vi "ShooterPID.vi"(9 "Shooter Refnum 2":string="My Motor RefNum", 10 "Shooter Refnum 1":string="My Motor RefNum") -> ()   [LabVIEW 2019]
uses:
  <vilib>/Rock Robotics/WPI/ThirdParty/REV Robotics/SPARK MAX/Typedef/Spark MAX Control Type.ctl
  sensors.vi
panel:
  in  "Setpoint Changer":dbl
  in  "Setpoint":dbl(slide) scale=-5700.0..5700.0
  out "PID Chart":T1(graph)
  in  "PID Constants":T2={"P Gain"=0.0012, "I Gain"=1e-06, "D Gain"=0.012, "F Gain"=0.00023, "I Zone"=100.0, "Min Output"=-1.0, "Max Output"=1.0} {"Max Output" min=-1.0 max=1.0 step=0.01; "Min Output" min=-1.0 max=1.0 step=0.01; "I Zone" step=0.01; "F Gain" step=0.01; "D Gain" step=0.01; "I Gain" step=0.01; "P Gain" min=0.0 step=0.01}
  in  "PID Constants 2":T2={"P Gain"=0.0012, "I Gain"=1e-06, "D Gain"=0.012, "F Gain"=0.00023, "I Zone"=100.0, "Min Output"=-1.0, "Max Output"=1.0} {"Max Output" min=-1.0 max=1.0 step=0.01; "Min Output" min=-1.0 max=1.0 step=0.01; "I Zone" step=0.01; "F Gain" step=0.01; "D Gain" step=0.01; "I Gain" step=0.01; "P Gain" min=0.0 step=0.01}
  out "PID Chart 2":T1(graph)
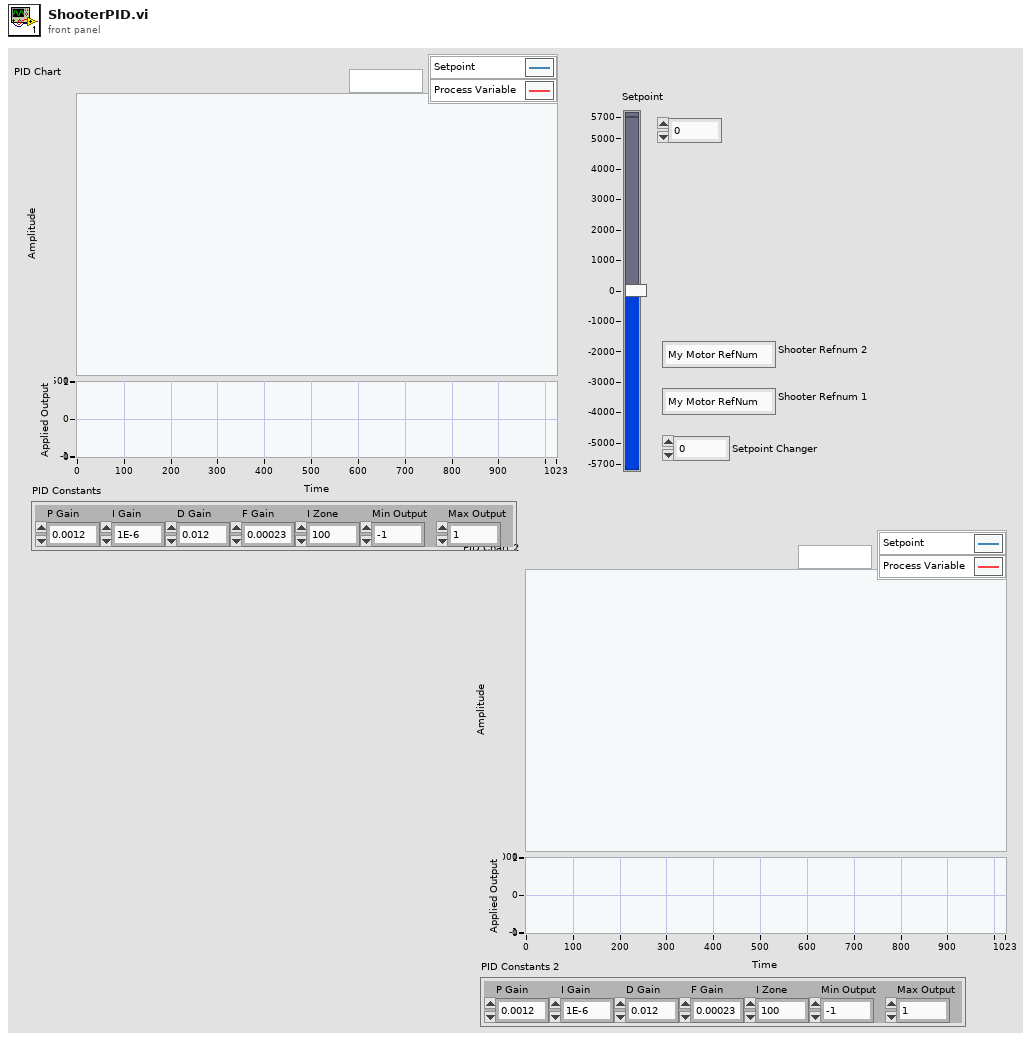
[diagram p1: front panel]
types:
  T1 = cluster{"Sensor Velocity":dbl, "Setpoint":dbl, "Applied Output":dbl}
  T2 = cluster{"P Gain":dbl, "I Gain":dbl, "D Gain":dbl, "F Gain":dbl, "I Zone":dbl, "Min Output":dbl, "Max Output":dbl}
  T3 = typedef "WPI_MotorControlDeviceRef.ctl" = cluster{"DeviceStatus":errorcluster, "Type":T4, "PWM":cluster{"PWM Channel":T5, "DeadBand":T6}, "CAN":cluster{"Device Number":u8, "SetOutput VI Ref":variant, "GetOutput VI Ref":variant, "Enable VI Ref":variant, "Disable VI Ref":variant, "Data":variant}, "Invert":bool, "DIO PWM":cluster{"PWM \"Enable\" Channel":T5, "DIOChannel":T7, "PWM Rate":dbl}}
  T4 = typedef "WPI_MotorControlType.ctl" = enum16{"PWM", "CAN", "DIO PWM"}
  T5 = typedef "FPGA_DIOPWMChannel.ctl" = enum8{"PWM 0", "PWM 1", "PWM 2", "PWM 3", "PWM 4", "PWM 5", "PWM 6", "PWM 7", "PWM 8", "PWM 9", "PWM MXP 0", "PWM MXP 1", "PWM MXP 2", "PWM MXP 3", "PWM MXP 4", "PWM MXP 5", "PWM MXP 6", "PWM MXP 7", "PWM MXP 8", "PWM MXP 9", "Invalid"}
  T6 = typedef "WPI_PWMDeadband.ctl" = cluster{"Name":string, "maxPositivePwm":i32, "minPositivePwm":i32, "centerPwm":i32, "maxNegativePwm":i32, "minNegativePwm":i32, "angularRange":u16}
  T7 = typedef "FPGA_DIOChannel.ctl" = enum8{"DIO 0", "DIO 1", "DIO 2", "DIO 3", "DIO 4", "DIO 5", "DIO 6", "DIO 7", "DIO 8", "DIO 9", "DIO MXP 0", "DIO MXP 1", "DIO MXP 2", "DIO MXP 3", "DIO MXP 4", "DIO MXP 5", "DIO MXP 6", "DIO MXP 7", "DIO MXP 8", "DIO MXP 9", "DIO MXP 10", "DIO MXP 11", "DIO MXP 12", "DIO MXP 13", "DIO MXP 14", "DIO MXP 15", "SPI Port CS1", "SPI Port CS2", "SPI Port CS3", "SPI Port MISO", "SPI Port MOSI", "Invalid"}
  T8 = typedef "Spark MAX Control Type.ctl" = enum16{"Percent VBus", "Voltage", "Velocity", "Position", "Smart Motion", "Current", "Smart Velocity"}
  T9 = cluster{"P Gain":bool, "I Gain":bool, "D Gain":bool, "F Gain":bool, "I Zone":bool, "Min Output":bool, "Max Output":bool}
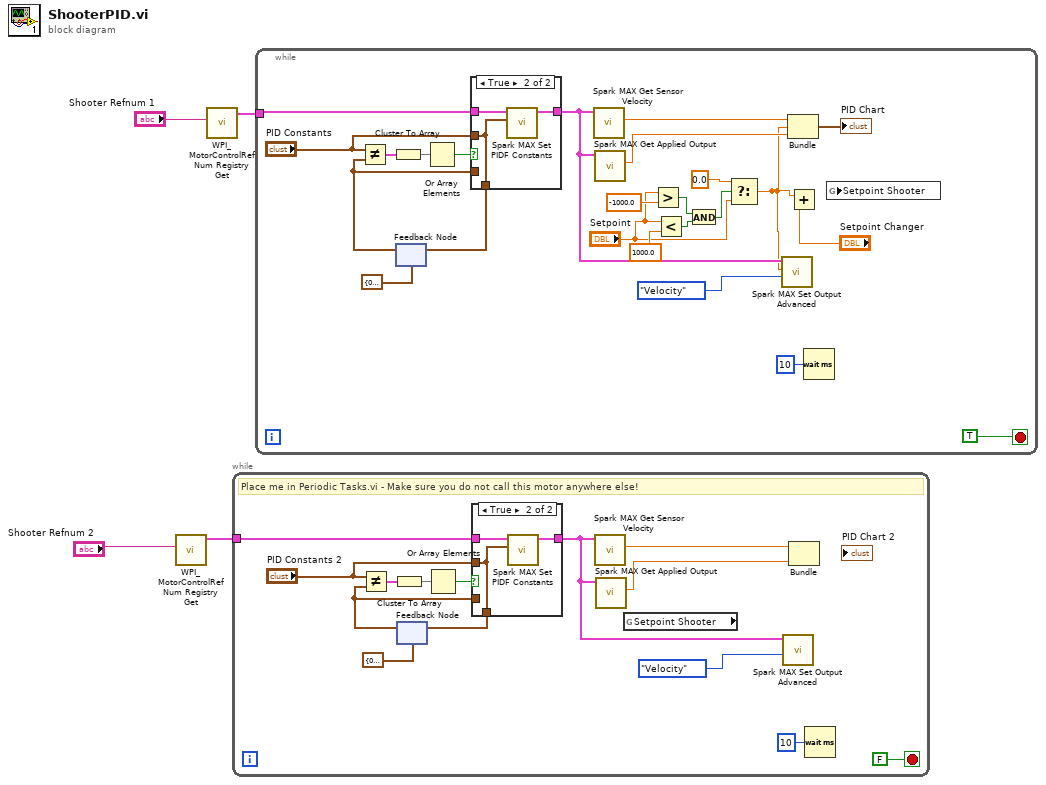
[diagram p0: block diagram]
diagram:
  n1 = call <vilib>:"WPI_MotorControlRefNum Registry Get.vi"("refnum name"="Shooter Refnum 2") -> ("MotorControlDevRef"=w4:T3)  [unwired: 9 in, 1 out]
  n2 = call <vilib>:"WPI_MotorControlRefNum Registry Get.vi"("refnum name"="Shooter Refnum 1") -> ("MotorControlDevRef"=w3:T3)  [unwired: 9 in, 1 out]
  n3 = while {
    tunnel: w4 -> [w5]
    stop <- FALSE stop-if-true
    # "Place me in Periodic Tasks.vi - Make sure you do not call this motor anywhere else!"
    n4 = feedback #1(T2 {"P Gain"=0.0, "I Gain"=0.0, "D Gain"=0.0, "F Gain"=0.0, "I Zone"=0.0, "Min Output"=0.0, "Max Output"=0.0} ("PID Constants")) -> (w17:T2)
    n5 = Not Equal?(x="PID Constants 2", y=w17) -> (x != y?=w11:T9)
    n6 = Cluster To Array(cluster=w11) -> (array=w12:bool[])
    n7 = Or Array Elements(Boolean array=w12) -> (logical OR=w14:bool)
    n8 = case shown="True" w14 {
      tunnel: w5 -> [w19 w23]
      tunnel: "PID Constants 2" -> [_ w21]
      tunnel: [w20 w21] -> w16
      tunnel: w17 -> [w20 _]
      tunnel: [w19 w22] -> w6
      frame False {
      }
      frame True {
        n9 = call <vilib>:"Spark MAX Set PIDF Constants.vi"("PID Constants"=w21, "MotorControlDeviceRef"=w23) -> ("MotorControlDeviceRef"=w22:T3)  [unwired: 8 in, 1 out]
      }
    }
    n10 = feedback-in #1(w16) -> ()
    n11 = call <vilib>:"Spark MAX Get Sensor Velocity.vi"("MotorControlDevRef in"=w6) -> ("Sensor Velocity"=w8:dbl)  [unwired: 7 in, 3 out]
    n12 = call <vilib>:"Spark MAX Get Applied Output.vi"("MotorControlDevRef in"=w6) -> ("Applied Output"=w7:dbl)  [unwired: 7 in, 3 out]
    n13 = global read "sensors.vi" "Setpoint Shooter"() -> ()  [unwired: 1 out]
    n14 = call <vilib>:"Spark MAX Set Output Advanced.vi"("Control Mode"=Spark_MAX_Control_Type."Velocity", "MotorControlDevRef"=w6) -> ()  [unwired: 8 in, 2 out]
    n15 = Bundle("Sensor Velocity"=w8, "Applied Output"=w7) -> ()  [unwired: 2 in, 1 out]
    n16 = Wait (ms)(milliseconds to wait=u32 10) -> ()  [unwired: 1 out]
  }
  n17 = while {
    tunnel: w3 -> [w25]
    stop <- TRUE stop-if-true
    n18 = feedback #2(T2 {"P Gain"=0.0, "I Gain"=0.0, "D Gain"=0.0, "F Gain"=0.0, "I Zone"=0.0, "Min Output"=0.0, "Max Output"=0.0} ("PID Constants")) -> (w45:T2)
    n19 = Not Equal?(x="PID Constants", y=w45) -> (x != y?=w39:T9)
    n20 = Cluster To Array(cluster=w39) -> (array=w40:bool[])
    n21 = Or Array Elements(Boolean array=w40) -> (logical OR=w42:bool)
    n22 = case shown="True" w42 {
      tunnel: "PID Constants" -> [_ w50]
      tunnel: [w48 w50] -> w44
      tunnel: w45 -> [w48 _]
      tunnel: [_ w51] -> w35
      tunnel: w25 -> [_ w49]
      frame False {
      }
      frame True {
        n23 = call <vilib>:"Spark MAX Set PIDF Constants.vi"("PID Constants"=w50, "MotorControlDeviceRef"=w49) -> ("MotorControlDeviceRef"=w51:T3)  [unwired: 8 in, 1 out]
      }
    }
    n24 = feedback-in #2(w44) -> ()
    n25 = call <vilib>:"Spark MAX Get Sensor Velocity.vi"("MotorControlDevRef in"=w35) -> ("Sensor Velocity"=w37:dbl)  [unwired: 7 in, 3 out]
    n26 = call <vilib>:"Spark MAX Get Applied Output.vi"("MotorControlDevRef in"=w35) -> ("Applied Output"=w36:dbl)  [unwired: 7 in, 3 out]
    n27 = Greater?(x="Setpoint", y=-1000.0) -> (0:w32:bool)
    n28 = Less?(x="Setpoint", y=1000.0) -> (x < y?=w31:bool)
    n29 = And(x=w32, y=w31) -> (x .and. y?=w30:bool)
    n30 = Select(t=0.0, s=w30, f="Setpoint") -> (s? t:f=w27:dbl)
    n31 = call <vilib>:"Spark MAX Set Output Advanced.vi"("Control Mode"=Spark_MAX_Control_Type."Velocity", "Setpoint"=w27, "MotorControlDevRef"=w35) -> ()  [unwired: 7 in, 2 out]
    n32 = Bundle("Sensor Velocity"=w37, "Setpoint"=w27, "Applied Output"=w36) -> (→"PID Chart":T1)  [unwired: 1 in]
    n33 = Add(x=w27, y="Setpoint Changer") -> ()  [unwired: 1 out]
    n34 = Wait (ms)(milliseconds to wait=u32 10) -> ()  [unwired: 1 out]
    n35 = global read "sensors.vi" "Setpoint Shooter"() -> ()  [unwired: 1 in]
  }
